vi "Read Flow Control.vi"(8 "error in (no error)":errorcluster, 11 "Serial Master in":refnum<class "Serial Master.lvclass">) -> (0 "error out":errorcluster, 2 "Flow Control":u16(ring) items=["None", "XON/XOFF", "RTS/CTS", "XON/XOFF & RTS/CTS", "DTR/DSR", "XON/XOFF & DTR/DSR"], 3 "Serial Master out":refnum<class "Serial Master.lvclass">)   [LabVIEW 2021, in "Serial Master.lvclass"]
uses:
  Serial Master.lvclass
  Serial Master.lvclass/Serial Master.ctl
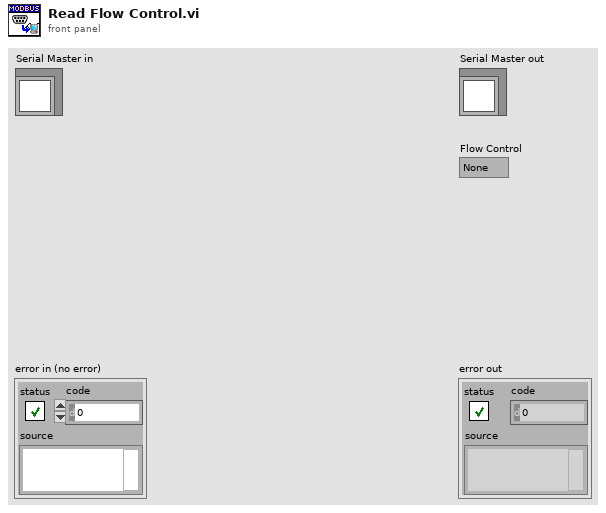
[diagram p1: front panel]
types:
  T1 = enum16{"None", "XON/XOFF", "RTS/CTS", "XON/XOFF & RTS/CTS", "DTR/DSR", "XON/XOFF & DTR/DSR"}
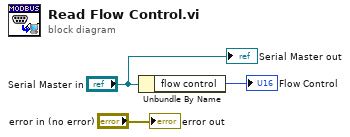
[diagram p0: block diagram]
diagram:
  n1 = Unbundle By Name("Serial Master in") -> ("flow control"=→"Flow Control":T1)
  "error out" <- "error in (no error)"
  "Serial Master out" <- "Serial Master in"
